vi "PLC触发信号分析.vi"(9 "队列集合输入":T1, 10 "上一次触发信号":bool[](array[boolean]), 11 "当前触发信号":bool[](array[boolean])) -> (3 "触发拍照":bool)   [LabVIEW 2014]
uses:
  Controls/PLCQueueOutput.ctl
  Controls/PLCQueueElement.ctl
  Controls/PLCAction.ctl
  Controls/Cam1QueueOutput.ctl
  Controls/Cam1QueueAction.ctl
  Controls/Cam2QueueAction.ctl
panel:
  out "触发信号上升沿":bool[](array[boolean])
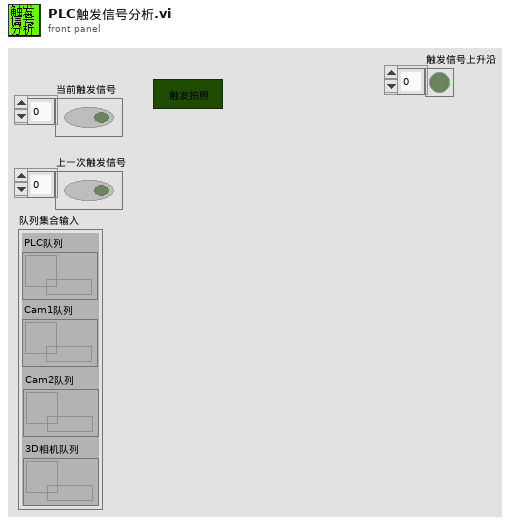
[diagram p1: front panel]
types:
  T1 = typedef "队列集合.ctl" = cluster{"PLC队列":T2, "Cam1队列":T3, "Cam2队列":refnum<queue>, "3D相机队列":refnum<queue>}
  T2 = typedef "PLCQueueOutput.ctl" = refnum<queue>
  T3 = typedef "Cam1QueueOutput.ctl" = refnum<queue>
  T4 = typedef "Cam1QueueAction.ctl" = enum16{"Cam1初始化", "Cam1待命", "Cam1预览", "Cam1手动", "Cam1自动"}
  T5 = typedef "Cam2QueueAction.ctl" = enum16{"Cam2初始化", "Cam2待命", "Cam2预览", "Cam2手动", "Cam2自动"}
  T6 = typedef "3D相机QueueAction.ctl" = enum16{"3D相机初始化", "3D相机待命", "3D相机预览", "3D相机手动", "3D相机自动"}
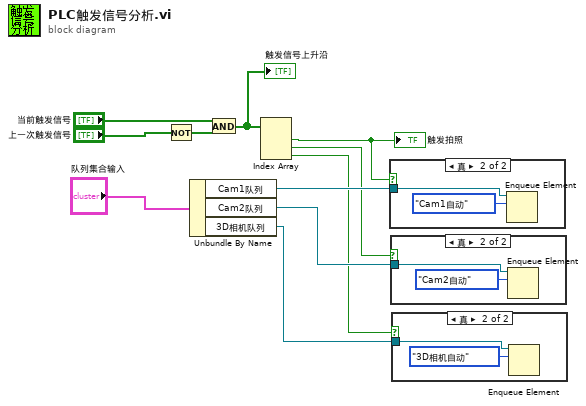
[diagram p0: block diagram]
diagram:
  n1 = Not(x="上一次触发信号") -> (.not. x?=w6:bool[])
  n2 = Unbundle By Name("队列集合输入") -> ("Cam1队列"=w10:T3, "Cam2队列"=w5:refnum<queue>, "3D相机队列"=w1:refnum<queue>)
  n3 = And(x="当前触发信号", y=w6) -> (x .and. y?=w8:bool[])
  "触发信号上升沿" <- w8
  n4 = Index Array(array=w8) -> (element #1=w4:bool, element #2=w3:bool, element #3=w2:bool)  [unwired: 3 in]
  "触发拍照" <- w4
  n5 = case shown="真" w4 {
    tunnel: w10 -> [_ w12]
    frame False {
    }
    frame True {
      n6 = Enqueue Element(queue=w12, element=Cam1QueueAction."Cam1自动" ("元素")) -> ()  [unwired: 2 in, 3 out]
    }
  }
  n7 = case shown="真" w3 {
    tunnel: w5 -> [_ w15]
    frame False {
    }
    frame True {
      n8 = Enqueue Element(queue=w15, element=Cam2QueueAction."Cam2自动" ("元素")) -> ()  [unwired: 2 in, 3 out]
    }
  }
  n9 = case shown="真" w2 {
    tunnel: w1 -> [_ w17]
    frame False {
    }
    frame True {
      n10 = Enqueue Element(queue=w17, element=3D相机QueueAction."3D相机自动" ("元素")) -> ()  [unwired: 2 in, 3 out]
    }
  }
